vi "API_Get_Directory_Tree.vi"() -> ()   [LabVIEW 2018]
uses:
  Controls/TekDriveSession.ctl
  <vilib>/httpClient/ClientHandle.ctl
  <vilib>/httpClient/LabVIEWHTTPClient.lvlib
panel:
  out "Error Out 2":errorcluster
  in  "Error In 2":errorcluster
  out "TekDrive Session 2":T1
  in  "TekDrive Session":T1
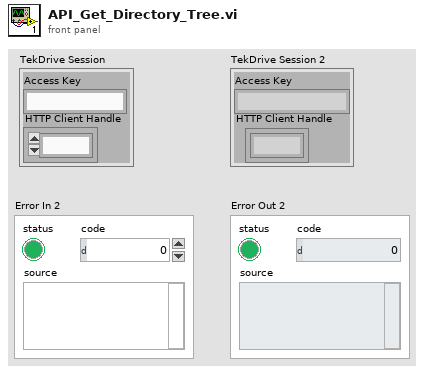
[diagram p1: front panel]
types:
  T1 = typedef "TekDriveSession.ctl" = cluster{"Access Key":string, "HTTP Client Handle":T2}
  T2 = typedef "LabVIEWHTTPClient.lvlib/ClientHandle.ctl" = refnum<k1>
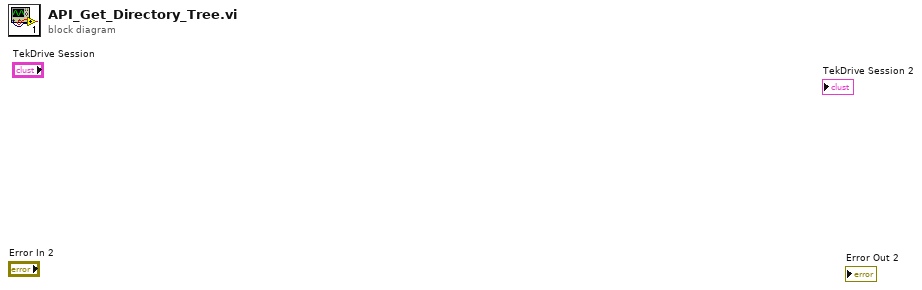
[diagram p0: block diagram]
diagram:
